vi "Test Basic Function 5.vi"() -> ()   [LabVIEW 2014]
uses:
  Arduino Math.lvlib
panel:
  out "lrint(x)":i32
  out "lround(x)":i32
  out "round(x)":sgl
  out "trunc(x)":sgl
  out "fmin(x,y)":sgl
  out "fmax(x,y)":sgl
  out "fma(x,y)":sgl
  out "pow(x,y) 2":sgl
  out "copysign(x,y)":sgl
  out "signbit(x)":i16
  out "inf? 2":bool
  out "inf?":bool
  out "NaN?":bool
  out "pow(x,y)":sgl
  out "log10(x)":sgl
  out "log(x)":sgl
  out "Error Out":errorcluster
  in  "Error In":errorcluster
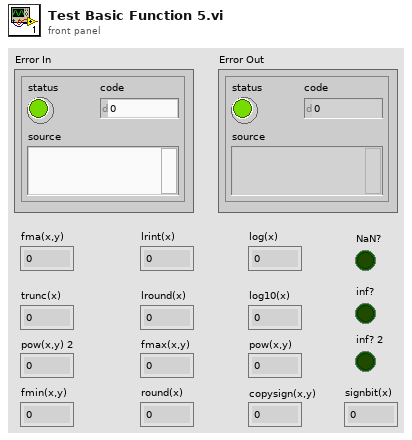
[diagram p1: front panel]
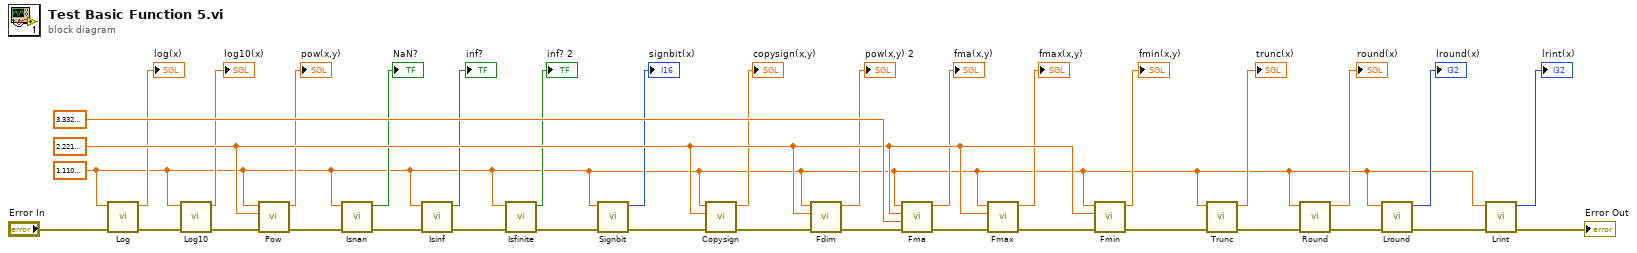
[diagram p0: block diagram]
diagram:
  w34 = sgl 2.222 ("x")
  w1 = sgl 1.111 ("x")
  n1 = call "Log.vi"("Error In"="Error In", "x"=w1) -> ("Error Out"=w33:errorcluster, "log(x)"=→"log(x)":sgl)  [unwired: 8 in]
  n2 = call "Log10.vi"("Error In"=w33, "x"=w1) -> ("Error Out"=w32:errorcluster, "log10(x)"=→"log10(x)":sgl)  [unwired: 8 in]
  n3 = call "Pow.vi"("Error In"=w32, "y"=w34, "x"=w1) -> ("Error Out"=w31:errorcluster, "pow(x,y)"=→"pow(x,y)":sgl)  [unwired: 7 in]
  n4 = call "Isnan.vi"("Error In"=w31, "x"=w1) -> ("Error Out"=w30:errorcluster, "NaN?"=→"NaN?":bool)  [unwired: 8 in]
  n5 = call "Isinf.vi"("Error In"=w30, "x"=w1) -> ("Error Out"=w29:errorcluster, "inf?"=→"inf?":bool)  [unwired: 8 in]
  n6 = call "Isfinite.vi"("Error In"=w29, "x"=w1) -> ("Error Out"=w28:errorcluster, "inf?"=→"inf? 2":bool)  [unwired: 8 in]
  n7 = call "Signbit.vi"("Error In"=w28, "x"=w1) -> ("Error Out"=w27:errorcluster, "signbit(x)"=→"signbit(x)":i16)  [unwired: 8 in]
  n8 = call "Copysign.vi"("Error In"=w27, "y"=w34, "x"=w1) -> ("Error Out"=w26:errorcluster, "copysign(x,y)"=→"copysign(x,y)":sgl)  [unwired: 7 in]
  n9 = call "Fdim.vi"("Error In"=w26, "y"=w34, "x"=w1) -> ("Error Out"=w25:errorcluster, "pow(x,y)"=→"pow(x,y) 2":sgl)  [unwired: 7 in]
  n10 = call "Fma.vi"("Error In"=w25, "z"=sgl 3.333 ("x"), "y"=w34, "x"=w1) -> ("Error Out"=w24:errorcluster, "fma(x,y)"=→"fma(x,y)":sgl)  [unwired: 6 in]
  n11 = call "Fmax.vi"("Error In"=w24, "y"=w34, "x"=w1) -> ("Error Out"=w23:errorcluster, "fmax(x,y)"=→"fmax(x,y)":sgl)  [unwired: 7 in]
  n12 = call "Fmin.vi"("Error In"=w23, "y"=w34, "x"=w1) -> ("Error Out"=w22:errorcluster, "fmin(x,y)"=→"fmin(x,y)":sgl)  [unwired: 7 in]
  n13 = call "Trunc.vi"("Error In"=w22, "x"=w1) -> ("Error Out"=w21:errorcluster, "trunc(x)"=→"trunc(x)":sgl)  [unwired: 8 in]
  n14 = call "Round.vi"("Error In"=w21, "x"=w1) -> ("Error Out"=w20:errorcluster, "round(x)"=→"round(x)":sgl)  [unwired: 8 in]
  n15 = call "Lround.vi"("Error In"=w20, "x"=w1) -> ("Error Out"=w4:errorcluster, "lround(x)"=→"lround(x)":i32)  [unwired: 8 in]
  n16 = call "Lrint.vi"("Error In"=w4, "x"=w1) -> ("Error Out"=→"Error Out":errorcluster, "lrint(x)"=→"lrint(x)":i32)  [unwired: 8 in]
